vi "HEWH SC3 Check Skip Condition.vi"(6 "Use Current Cond?":bool, 8 "Error In":errorcluster, 9 "Saved Condition":T1, 10 "Condition#":T1, 11 "Current Cond":T1) -> (0 "Error Out":errorcluster, 2 "Conditions Equal?":bool, 3 "SC3 Check Skip":T1)   [LabVIEW 2019]
uses:
  Type Definitions/HEWH Special Condition Check.ctl
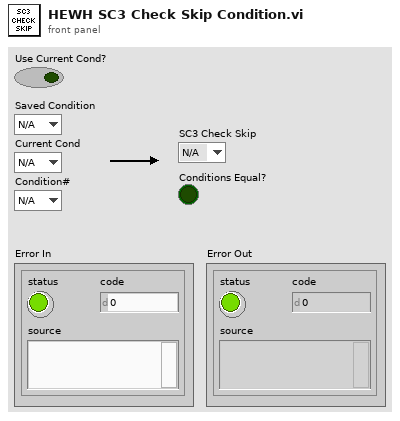
[diagram p1: front panel]
types:
  T1 = typedef "HEWH Special Condition Check.ctl" = enum16{"N/A", "C1", "C2", "Reset/Fail", "Skip Draw Sequence"}
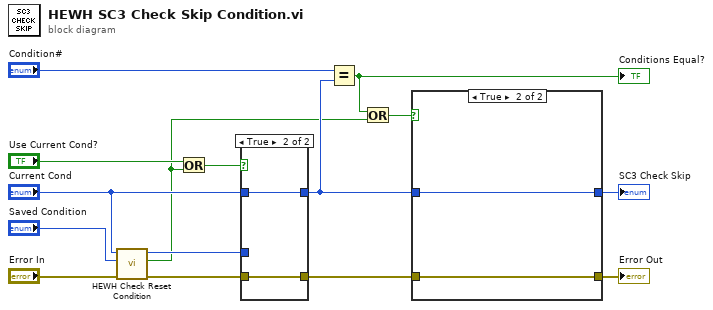
[diagram p0: block diagram]
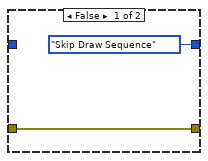
[diagram p3: hidden frame]
diagram:
  n1 = call "HEWH Check Reset Condition.vi"("Error In"="Error In", "SC3 Check Skip"="Saved Condition", "Current Cond"="Current Cond") -> ("Error Out"=w7:errorcluster, "Equals Reset Fail?"=w2:bool, "Current Cond"=w9:T1)  [unwired: 6 in]
  n2 = Or(x="Use Current Cond?", y=w2) -> (x .or. y?=w4:bool)
  n3 = case shown="True" w4 {
    tunnel: [w17 w19] -> w12
    tunnel: "Current Cond" -> [_ w19]
    tunnel: w9 -> [w17 _]
    tunnel: w7 -> [w16 w18]
    tunnel: [w16 w18] -> w6
    frame False {
    }
    frame True {
    }
  }
  n4 = Equal?(x="Condition#", y=w12) -> (x = y?=w3:bool)
  "Conditions Equal?" <- w3
  n5 = Or(x=w3, y=w2) -> (x .or. y?=w1:bool)
  n6 = case shown="True" w1 {
    tunnel: [HEWH_Special_Condition_Check."Skip Draw Sequence" ("Special Cond Seq") w23] -> w14
    tunnel: w12 -> [_ w23]
    tunnel: w6 -> [w20 w22]
    tunnel: [w20 w22] -> w13
    frame False {
    }
    frame True {
    }
  }
  "SC3 Check Skip" <- w14
  "Error Out" <- w13
